vi "NewtonsPPA_Meas_Scope.vi"(0 "VISA session":refnum<visa-resource-name>, 7 "Phase Selection (Phase 1)":u16(ring) items=["Phase 1", "Phase 2", "Phase 3", "Neutral"], 9 "Measurement Type (Voltage)":u16(ring) items=["Voltage", "Current"], 11 "error in (no error)":errorcluster) -> (4 "dup VISA session":refnum<visa-resource-name>, 6 "Read Strings":string, 8 "Waveform":dbl[][](graph), 15 "error out":errorcluster)   [LabVIEW 2025, in "NewtonsPSM1735.lvlib"]
doc: "This VI reads the scope data from the PPA2530"
uses:
  NewtonsPSM1735.lvlib
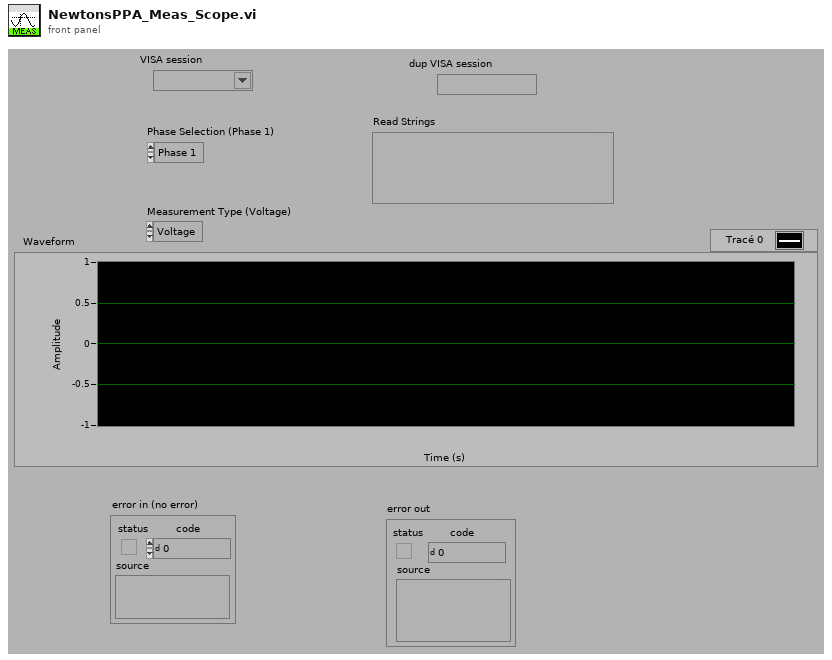
[diagram p1: front panel]
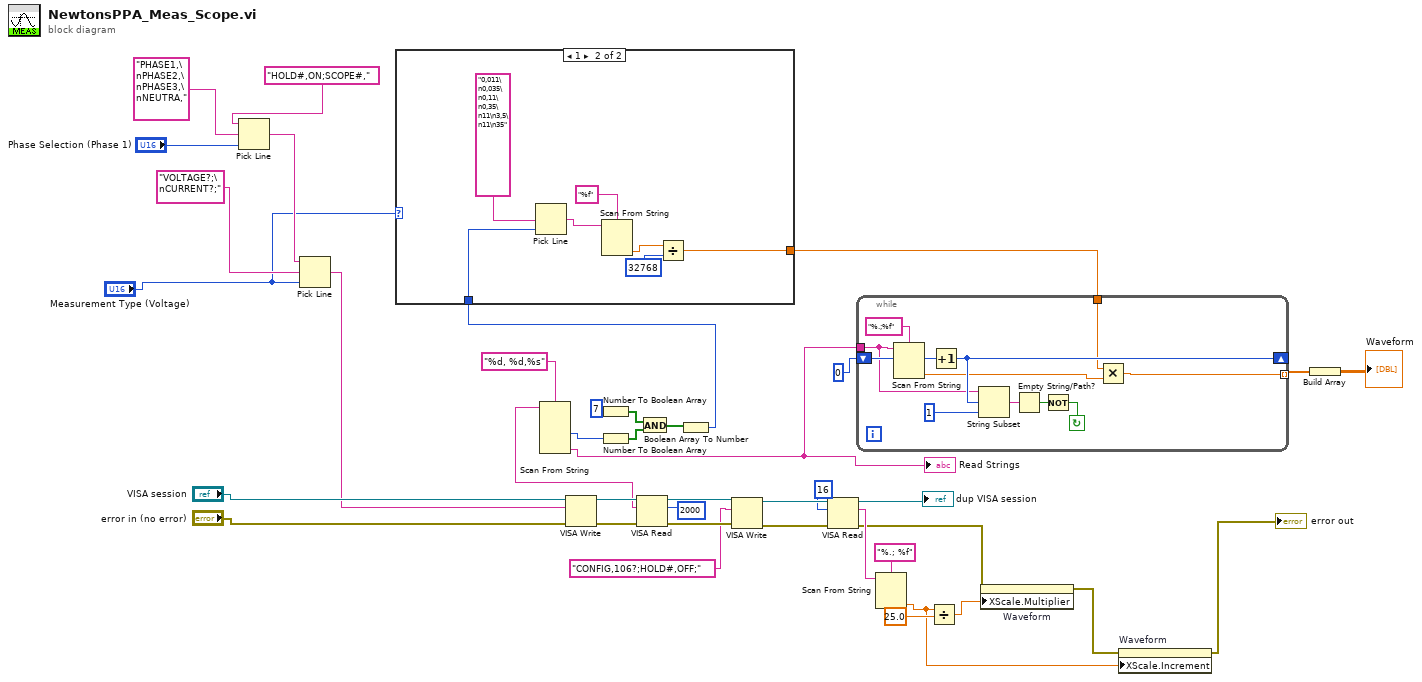
[diagram p0: block diagram]
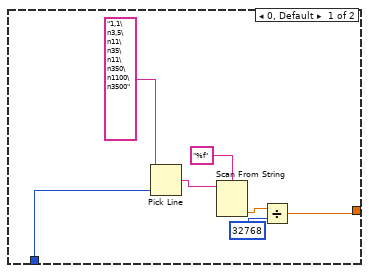
[diagram p2: hidden frame]
diagram:
  n1 = Pick Line(string ("")="HOLD#,ON;SCOPE#,", multi-line string="PHASE1,\nPHASE2,\nPHASE3,\nNEUTRA,", line index="Phase Selection (Phase 1)") -> (output string=w37:string)
  n2 = Pick Line(string ("")=w37, multi-line string="VOLTAGE?;\nCURRENT?;", line index="Measurement Type (Voltage)") -> (output string=w25:string)
  n3 = VISA Write(VISA resource name="VISA session", write buffer=w25, error in (no error)="error in (no error)") -> (VISA resource name out=w34:refnum<visa-resource-name>, error out=w33:errorcluster)  [unwired: 1 out]
  n4 = Number To Boolean Array(number=7) -> (Boolean array=w19:bool[])
  n5 = VISA Read(VISA resource name=w34, byte count=u32 2000 ("ÊÞ²Ä¶³ÝÄi0j"), error in (no error)=w33) -> (VISA resource name out=w14:refnum<visa-resource-name>, read buffer=w24:string, error out=w15:errorcluster)  [unwired: 1 out]
  n6 = Scan From String(format string="%d, %d,%s" ("chaîne de format"), input string=w24) -> (output 1=w21:i32, output 3=w22:string)  [unwired: 2 in, 7 out]
  "Read Strings" <- w22
  n7 = Number To Boolean Array(number=w21) -> (Boolean array=w18:bool[])
  n8 = And(x=w19, y=w18) -> (x .and. y?=w17:bool[])
  n9 = Boolean Array To Number(Boolean array=w17) -> (number=w16:u32)
  n10 = case shown="1" "Measurement Type (Voltage)" {
    tunnel: [w42 w50] -> w28
    tunnel: w16 -> [w41 w48]
    frame 0, Default {
      n11 = Pick Line(multi-line string="1,1\n3,5\n11\n35\n11\n350\n1100\n3500", line index=w41) -> (output string=w45:string)  [unwired: 1 out]
      n12 = Scan From String(format string="%f" ("chaîne de format"), input string=w45) -> (output 1=w43:dbl)  [unwired: 2 in, 4 out]
      n13 = Divide(x=w43, y=32768) -> (x/y=w42:dbl)
    }
    frame 1 {
      n14 = Pick Line(multi-line string="0,011\n0,035\n0,11\n0,35\n11\n3,5\n11\n35", line index=w48) -> (output string=w52:string)  [unwired: 1 out]
      n15 = Scan From String(format string="%f" ("chaîne de format"), input string=w52) -> (output 1=w51:dbl)  [unwired: 2 in, 4 out]
      n16 = Divide(x=w51, y=32768) -> (x/y=w50:dbl)
    }
  }
  n17 = VISA Write(VISA resource name=w14, write buffer="CONFIG,106?;HOLD#,OFF;", error in (no error)=w15) -> (VISA resource name out=w13:refnum<visa-resource-name>, error out=w12:errorcluster)  [unwired: 1 out]
  n18 = VISA Read(VISA resource name=w13, byte count=16, error in (no error)=w12) -> (VISA resource name out=→"dup VISA session":refnum<visa-resource-name>, read buffer=w8:string, error out=w2:errorcluster)  [unwired: 1 out]
  n19 = while {
    tunnel: [w57] -> w30 mode=indexing
    shift-left: 0 -> [w59]
    shift-right: [w62] -> _
    tunnel: w28 -> [w56]
    tunnel: w22 -> [w55]
    stop <- w63 continue-if-true
    n20 = Scan From String(format string="%.;%f", input string=w55, initial scan location=w59) -> (offset past scan=w60:u32, output 1=w58:dbl)  [unwired: 1 in, 3 out]
    n21 = Increment(x=w60) -> (x+1=w62:u32)
    n22 = String Subset(string=w55, offset (0)=w62, length (rest)=1) -> (substring=w65:string)
    n23 = Empty String/Path?(string/path=w65) -> (empty?=w64:bool)
    n24 = Not(x=w64) -> (.not. x?=w63:bool)
    n25 = Multiply(x=w56, y=w58) -> (x*y=w57:dbl)
  }
  n26 = Scan From String(format string="%.; %f" ("chaîne de format"), input string=w8) -> (output 1=w4:dbl)  [unwired: 2 in, 4 out]
  n27 = Divide(x=w4, y=25.0) -> (x/y=w6:dbl)
  n28 = property on="Waveform" class="WFGraph (strict)"(error in=w2, "XScale.Multiplier"=w6) -> (error out=w3:errorcluster)  [unwired: 1 in, 1 out]
  n29 = property on="Waveform" class="WFGraph (strict)"(error in=w3, "XScale.Increment"=w4) -> (error out=→"error out":errorcluster)  [unwired: 1 in, 1 out]
  n30 = Build Array(w30) -> (→"Waveform":dbl[][])
